vi "Get Context by ID.vi"(8 "Error In":errorcluster, 10 "Sequence ID":i32, 11 "Application Manager":refnum<k7>) -> (0 "Error Out":errorcluster, 3 "Sequence Context":refnum<k7>)   [LabVIEW 2021, in "Seq Edit Quick Drop.lvlib"]
uses:
  Seq Edit Quick Drop.lvlib
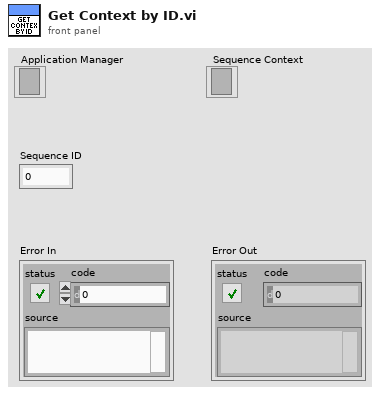
[diagram p1: front panel]
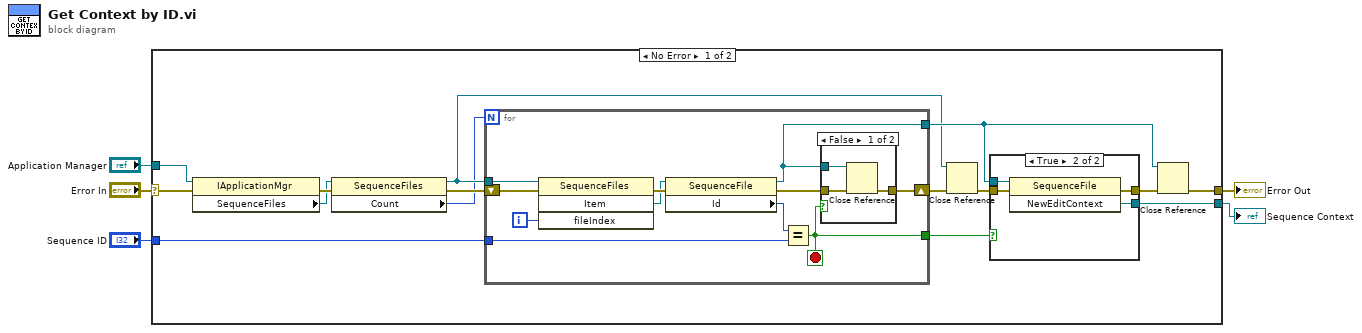
[diagram p0: block diagram]
diagram:
  n1 = case shown="No Error" "Error In" {
    selector: "Error In" -> [w7 w41]
    tunnel: "Sequence ID" -> [w17 _]
    tunnel: "Application Manager" -> [w12 _]
    tunnel: [w11 _] -> w3
    tunnel: [w8 w41] -> w2
    frame No Error {
      n2 = property class="IApplicationMgr"(reference=w12, error in=w7) -> (error out=w20:errorcluster, "SequenceFiles"=w19:refnum<k7>)  [unwired: 1 out]
      n3 = property class="SequenceFiles"(reference=w19, error in=w20) -> (reference out=w9:refnum<k7>, error out=w18:errorcluster, "Count"=w6:i32)
      n4 = for {
        N: w6 -> [_]
        shift-right: [w28] -> w15
        shift-left: w18 -> [w33]
        tunnel: w9 -> [w32]
        tunnel: w17 -> [w29]
        tunnel: [w26] -> w13
        tunnel: [w27] -> w16
        i -> [w35]
        stop <- w27 stop-if-true
        n5 = invoke class="SequenceFiles" method="Item"(reference=w32, error in=w33, "fileIndex"=w35) -> (error out=w36:errorcluster, "Item"=w34:refnum<k7>)  [unwired: 1 in, 2 out]
        n6 = property class="SequenceFile"(reference=w34, error in=w36) -> (reference out=w26:refnum<k7>, error out=w31:errorcluster, "Id"=w30:i32)
        n7 = Equal?(x=w30, y=w29) -> (x = y?=w27:bool)
        n8 = case shown="False" w27 {
          tunnel: w31 -> [w39 w40]
          tunnel: [w38 w40] -> w28
          tunnel: w26 -> [w37 _]
          frame False {
            n9 = Close Reference(reference=w37, error in (no error)=w39) -> (error out=w38:errorcluster)
          }
          frame True {
          }
        }
      }
      n10 = Close Reference(reference=w9, error in (no error)=w15) -> (error out=w10:errorcluster)
      n11 = case shown="True" w16 {
        tunnel: w13 -> [_ w25]
        tunnel: w10 -> [w21 w24]
        tunnel: [w21 w23] -> w14
        tunnel: [_ w22] -> w11
        frame False {
        }
        frame True {
          n12 = invoke class="SequenceFile" method="NewEditContext"(reference=w25, error in=w24) -> (error out=w23:errorcluster, "NewEditContext"=w22:refnum<k7>)  [unwired: 1 in, 1 out]
        }
      }
      n13 = Close Reference(reference=w13, error in (no error)=w14) -> (error out=w8:errorcluster)
    }
    frame Error {
    }
  }
  "Error Out" <- w2
  "Sequence Context" <- w3
